vi "Send to Tulip.vi"(8 "Data file name":string, 9 "Result":string, 11 "Serial number":string) -> (0 "error out":errorcluster, 1 "Status String":string, 3 "Response body":string)   [LabVIEW 2021]
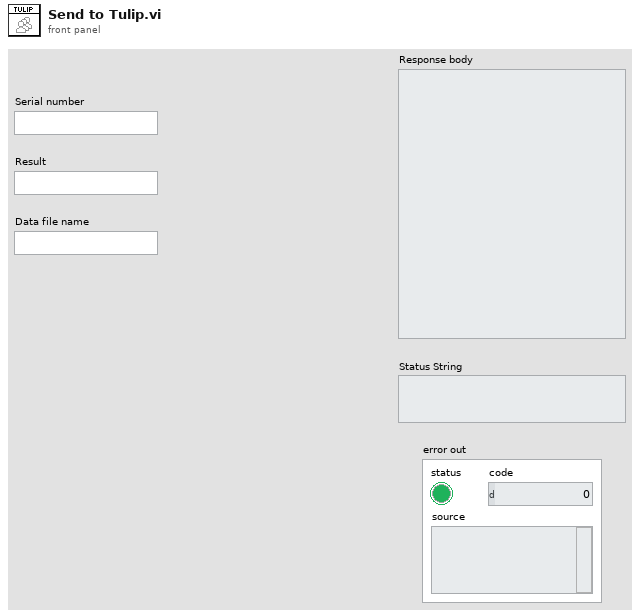
[diagram p1: front panel]
types:
  T1 = cluster{"id":string, "qexvc_serial_number":string, "lytqu_parameter":string, "oebrh_result":string, "ogkyt_date":string, "tjuiw_data_file":string}
  T2 = enum16{"Init", "Get headers", "Get", "Post", "Put", "Close"}
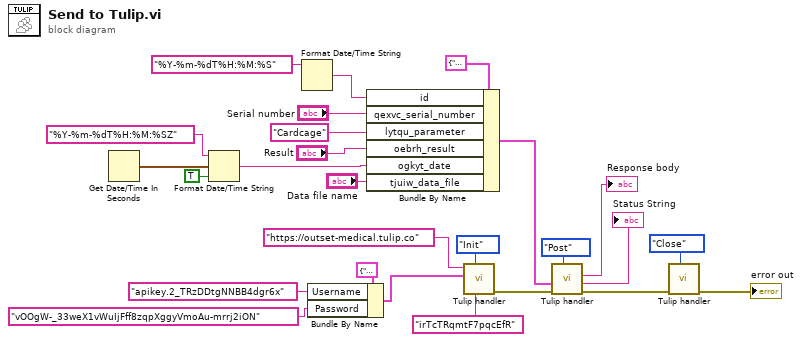
[diagram p0: block diagram]
diagram:
  n1 = Get Date/Time In Seconds() -> (seconds since 1Jan1904=w11:timestamp)
  n2 = Format Date/Time String(time format string (%c)="%Y-%m-%dT%H:%M:%SZ", seconds (now)=w11, UTC format=TRUE) -> (date/time string=w5:string)
  n3 = Format Date/Time String(time format string (%c)="%Y-%m-%dT%H:%M:%S") -> (date/time string=w6:string)  [unwired: 2 in]
  n4 = Bundle By Name(cluster=cluster{"Username":string, "Password":string} {"Username"="apikey.2_WNWgDzkcRL7LwQrSC", "Password"="uUTRYqQF2kxie-OG2NdFiDN_Ok5rwnamrdCqWvd0OVz"} ("Authentication"), "Username"="apikey.2_TRzDDtgNNBB4dgr6x", "Password"="vOOgW-_33weX1vWuIjFff8zqpXggyVmoAu-mrrj2iON") -> (w23:cluster{"Username":string, "Password":string})
  n5 = Bundle By Name(cluster=T1 {"id"="", "qexvc_serial_number"="", "lytqu_parameter"="", "oebrh_result"="", "ogkyt_date"="", "tjuiw_data_file"=""} ("Body"), "id"=w6, "qexvc_serial_number"="Serial number", "lytqu_parameter"="Cardcage", "oebrh_result"="Result", "ogkyt_date"=w5, "tjuiw_data_file"="Data file name") -> (w1:T1)
  n6 = call "Tulip handler.vi"("Table ID"="irTcTRqmtF7pqcEfR", "State"=T2."Init", "Authentication"=w23, "URL"="https://outset-medical.tulip.co") -> ("error out"=w26:errorcluster)  [unwired: 5 in, 2 out]
  n7 = call "Tulip handler.vi"("State"=T2."Post", "error in"=w26, "Body"=w1) -> ("error out"=w17:errorcluster, "Status String"=→"Status String":string, "Response body"=→"Response body":string)  [unwired: 6 in]
  n8 = call "Tulip handler.vi"("State"=T2."Close", "error in"=w17) -> ("error out"=→"error out":errorcluster)  [unwired: 7 in, 2 out]
